vi "17_SoftwareClock.vi"() -> ()   [LabVIEW 2014]
uses:
  SwabianInstruments.TimeTagger
panel:
  out "SoftwareClockState":T1={"enabled"=FALSE, "is_locked"=FALSE, "period_error"=nan, "phase_error_estimation"=nan, "clock_period"=0, "error_counter"=0}
  in  "SoftwareClock settings":T2={"clock source"=enum."test signal as external clock", "input freq."=900000.0, "averaging_periods"=100.0, "trace_len"=1000, "clock channel"=1}
  in  "FrequencyStability settings":T3={"average"=1, "steps start"=1, "steps end"=100000, "number of steps"=100, "signal source"=enum."test signal", "signal channel"=2} {"number of steps" min=2 max=1000}
  out "Frequency error":T4(graph)
  out "Phase error":T5(graph)
  out "logger output":string="########################\n\nThis example demonstrates the SoftwareClock. The SoftwareClock is the recommended way to apply an external clock to the Time Tagger. Here, we will use the internal test signal for demonstration purposes. Be aware that this means decreasing the quality of the internal clock of your Time Tagger! If you have a high-quality external reference available, feel free to apply this and to set \"clock source\" to \"external clock\".\n\nThe settings of the SoftwareClock are updated every when the measurement is started.\n\nThe FrequencyStability measurement class provides numerous standard metrics conforming to IEEE 1139, e.g. the Allan Deviation (ADEV).\n\n########################\r\n\r\n"
  in  "exit":bool
  in  "run measurement":bool
  out "Time domain":cluster{"getTau":dbl[], "getHDEV":dbl[]}[](graph)
  out "Allan domain":cluster{"getTau":dbl[], "getSTDD":dbl[]}[](graph)
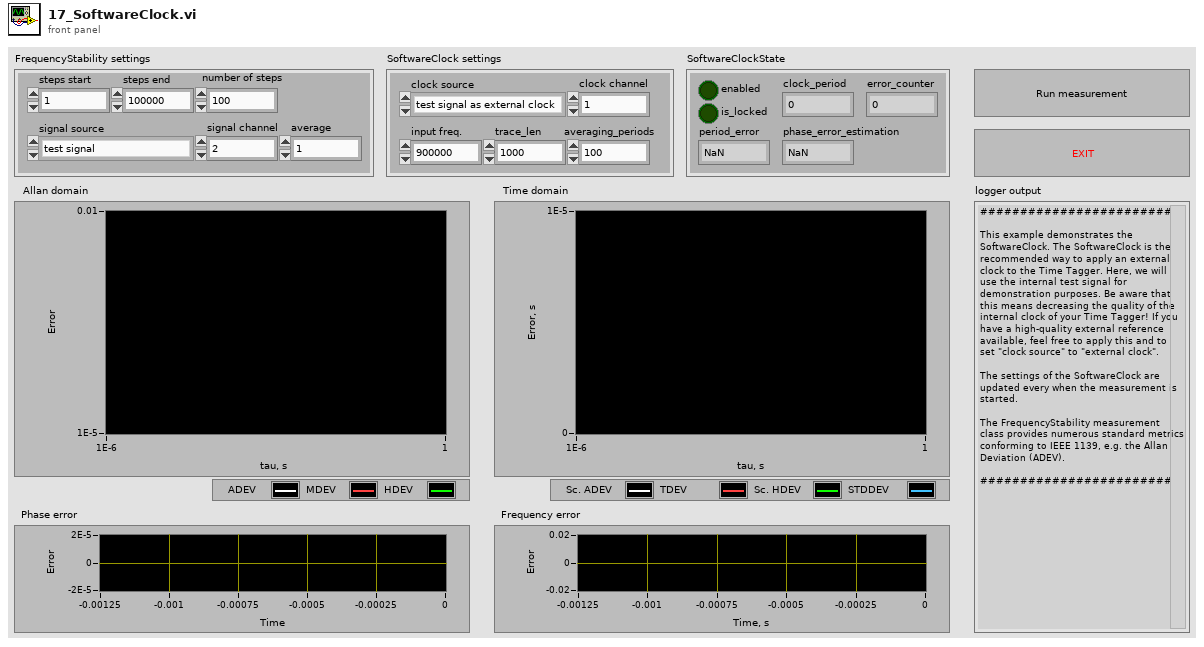
[diagram p1: front panel]
types:
  T1 = cluster{"enabled":bool, "is_locked":bool, "period_error":dbl, "phase_error_estimation":dbl, "clock_period":i64, "error_counter":i64}
  T2 = cluster{"clock source":enum16{"internal clock", "external clock", "test signal as external clock"}, "input freq.":dbl, "averaging_periods":dbl, "trace_len":u64, "clock channel":i32}
  T3 = cluster{"average":i64, "steps start":i32, "steps end":i32, "number of steps":i32, "signal source":enum16{"external signal", "test signal"}, "signal channel":i32}
  T4 = cluster{"getTraceIndex":dbl[], "getTraceFrequency":dbl[]}
  T5 = cluster{"getTraceIndex":dbl[], "getTracePhase":dbl[]}
  T6 = enum16{"internal clock", "external clock", "test signal as external clock"}
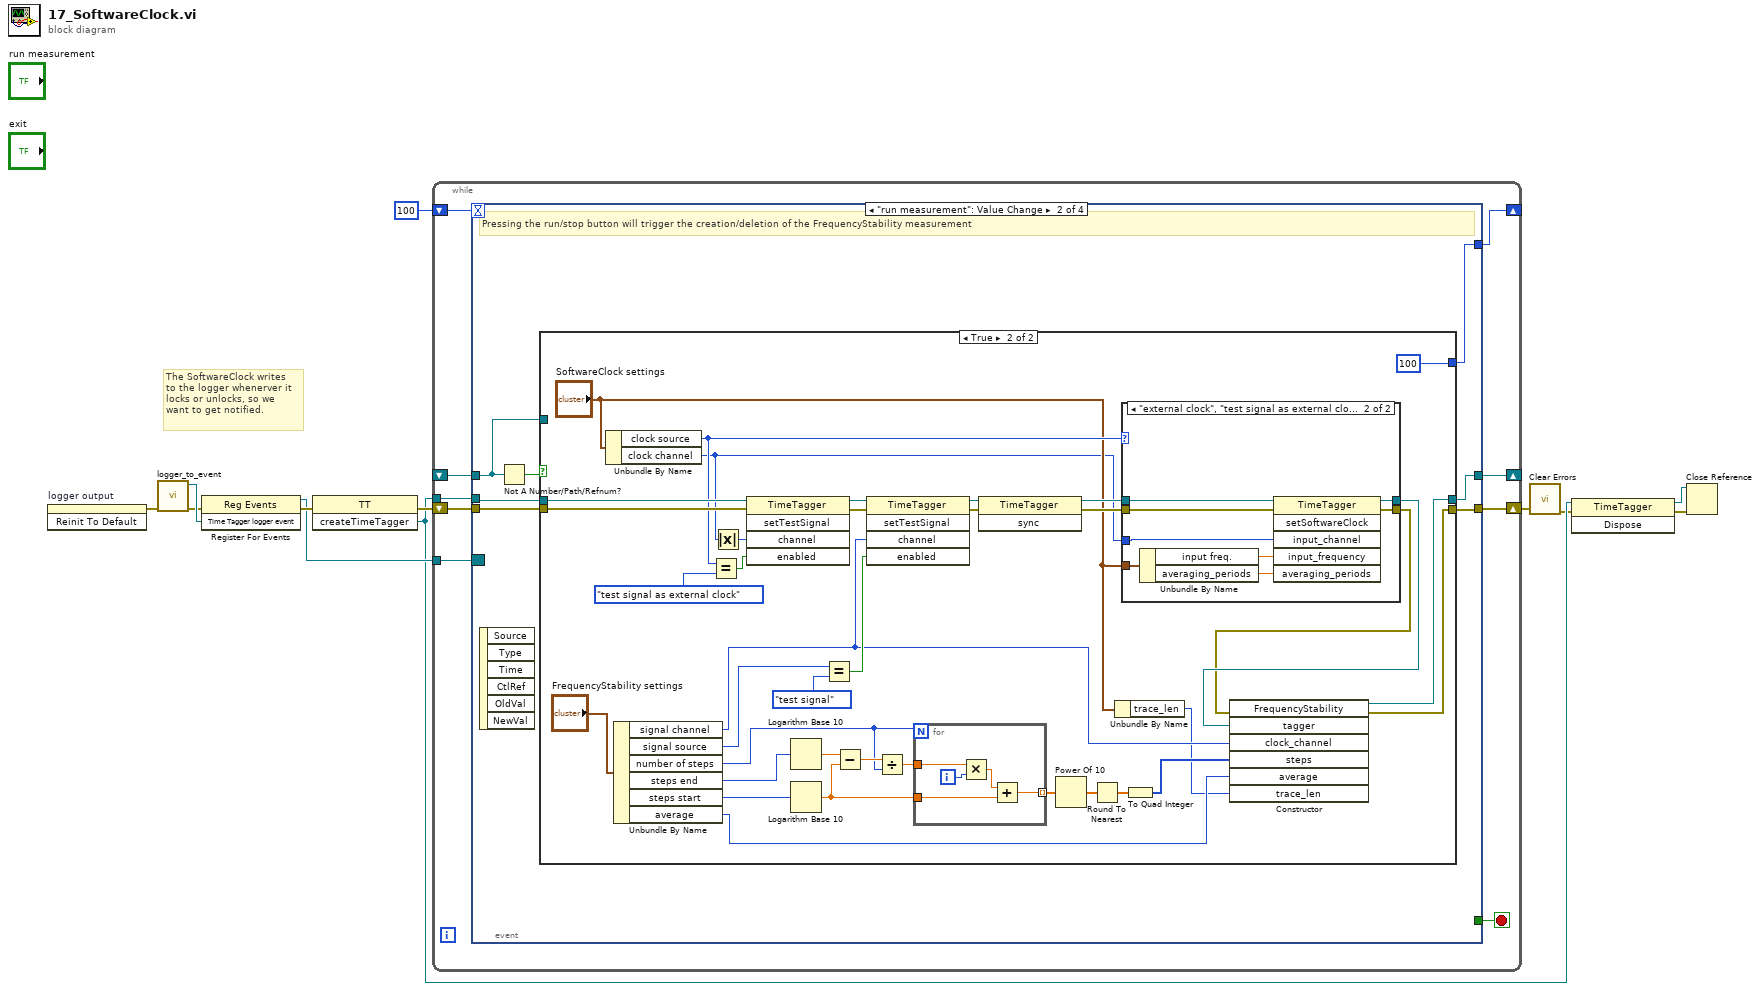
[diagram p0: block diagram]
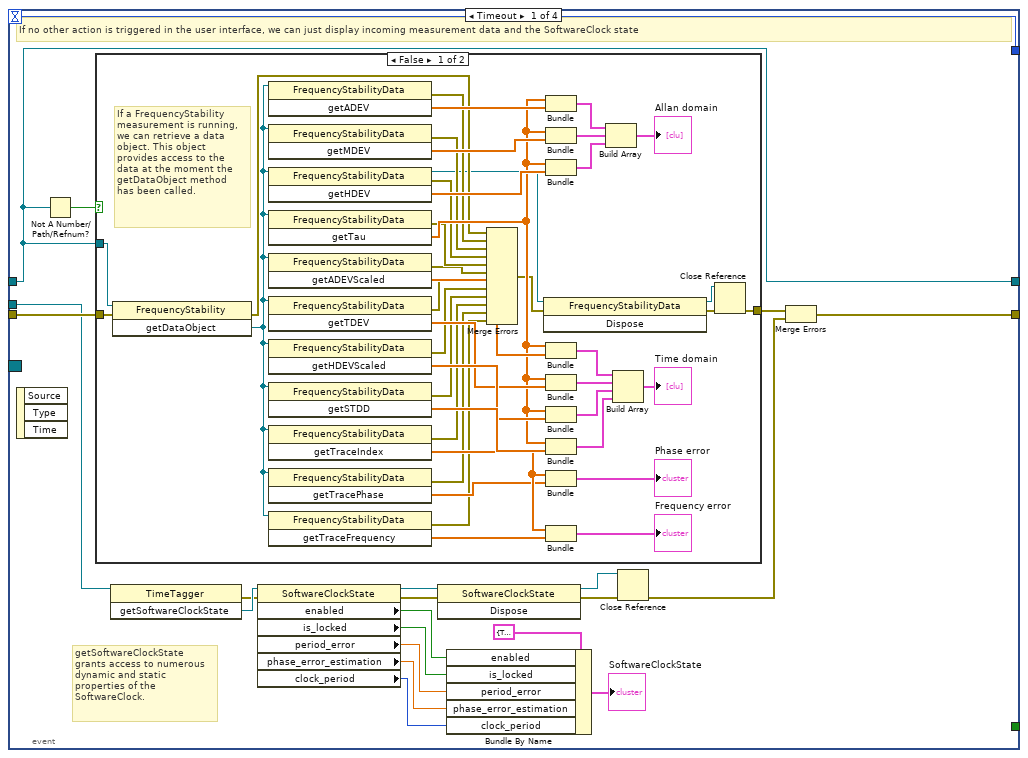
[diagram p2: hidden frame]
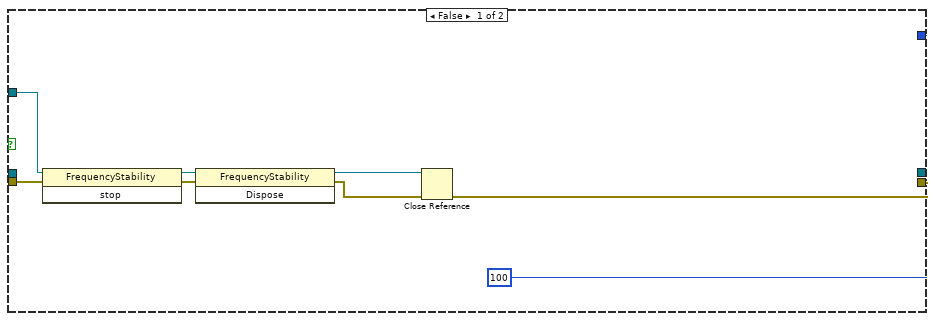
[diagram p4: hidden frame]
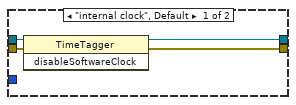
[diagram p5: hidden frame]
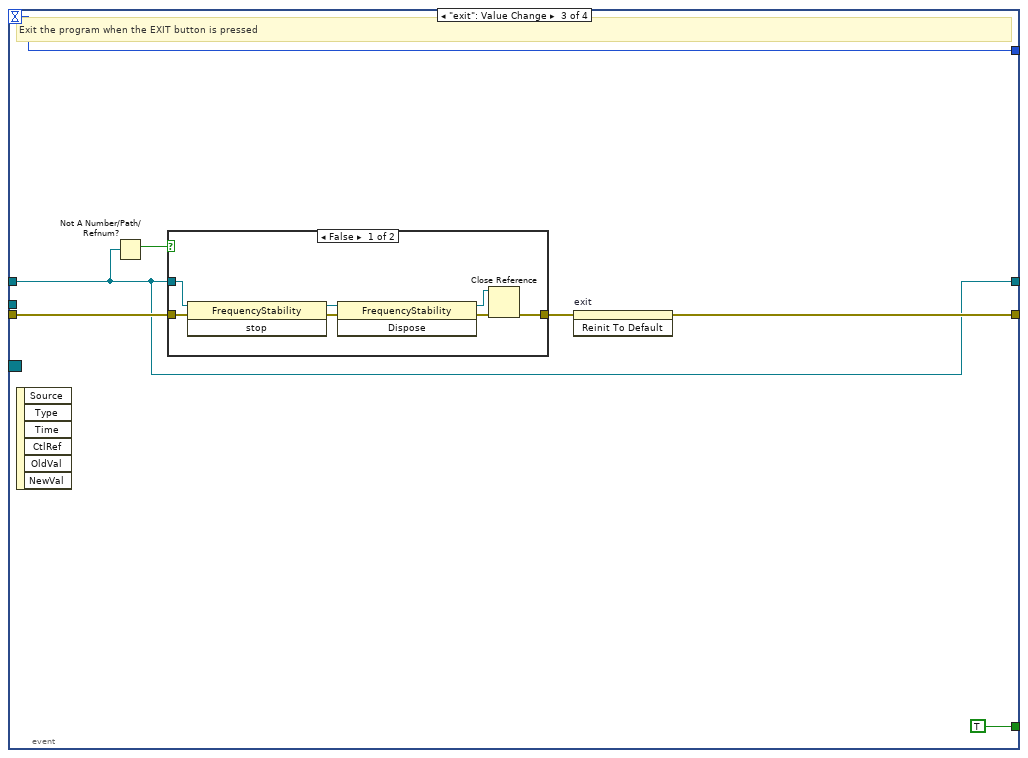
[diagram p6: hidden frame]
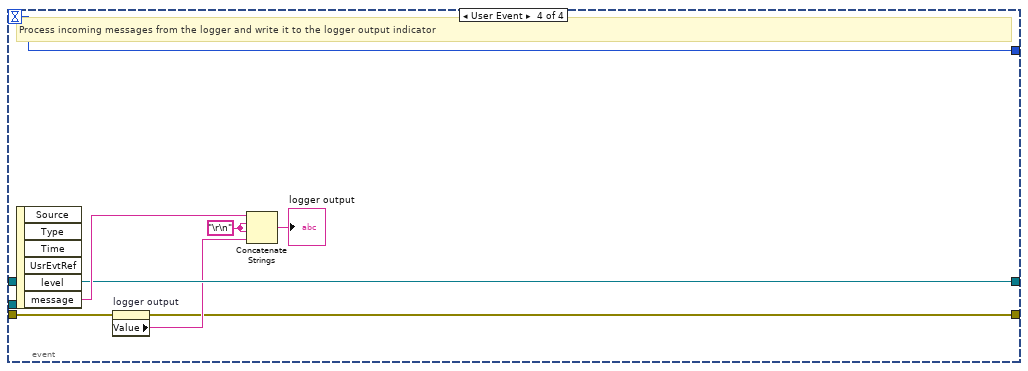
[diagram p8: hidden frame]
diagram:
  # "The SoftwareClock writes\nto the logger whenerver it\nlocks or unlocks, so we\nwant to get notified."
  n1 = invoke on="logger output" class="Str" method="Reinit To Default"() -> (error out=w6:errorcluster)  [unwired: 3 in, 2 out]
  n2 = call "logger_to_event.vi"("error in (no error)"=w6) -> ("error out"=w9:errorcluster, "Time Tagger logger event"=w10:refnum<user-event>)  [unwired: 9 in]
  n3 = register-events(error in=w9, w10) -> (reference out=w7:refnum<event-registration>, error out=w8:errorcluster)  [unwired: 1 in]
  n4 = invoke class="TT" method="createTimeTagger"(error in=w8) -> (error out=w11:errorcluster, "createTimeTagger"=w4:refnum<k24>)  [unwired: 2 in, 1 out]
  n5 = while {
    tunnel: w4 -> [w21]
    shift-right: [w20] -> _
    shift-left: _ -> [w19]
    shift-right: [w17] -> _
    shift-left: 100 -> [w18]
    shift-right: [w15] -> w5
    shift-left: w11 -> [w16]
    tunnel: w7 -> [w13]
    stop <- w14 stop-if-true
    n6 = event shown="[1] \"run measurement\": Value Change" {
      selector: w13 -> [_ _ _ _]
      dyn-events: _ -> [_ _ _ _]
      timeout: w18 -> [w25 _ w159 w175]
      tunnel: w21 -> [w40 w92 _ _]
      tunnel: [w42 w91 w155 w176] -> w20
      tunnel: w19 -> [w42 w89 w155 w176]
      tunnel: [w25 w88 w159 w175] -> w17
      tunnel: w16 -> [w41 w87 w156 w170]
      tunnel: [w23 w86 w161 w171] -> w15
      tunnel: [_ _ TRUE _] -> w14
      event Timeout {
        # "getSoftwareClockState\ngrants access to numerous\ndynamic and static\nproperties of the\nSoftwareClock."
        # "If no other action is triggered in the user interface, we can just display incoming measurement data and the SoftwareClock state"
        n7 = event-data() -> ()  [unwired: 1 in, 3 out]
        n8 = Not A Number/Path/Refnum?(number/path/refnum=w42) -> (NaN/Path/Refnum?=w39:bool)
        n9 = case shown="False" w39 {
          tunnel: w42 -> [w84 _]
          tunnel: w41 -> [w83 w85]
          tunnel: [w61 w85] -> w24
          frame False {
            # "If a FrequencyStability\nmeasurement is running,\nwe can retrieve a data\nobject. This object\nprovides access to the\ndata at the moment the\ngetDataObject method\nhas been called."
            n10 = invoke class="FrequencyStability" method="getDataObject"(reference=w84, error in=w83) -> (error out=w65:errorcluster, "getDataObject"=w60:refnum<k24>)  [unwired: 1 in, 1 out]
            n11 = invoke class="FrequencyStabilityData" method="getADEV"(reference=w60) -> (error out=w54:errorcluster, "getADEV"=w82:dbl[])  [unwired: 2 in, 1 out]
            n12 = invoke class="FrequencyStabilityData" method="getMDEV"(reference=w60) -> (error out=w53:errorcluster, "getMDEV"=w81:dbl[])  [unwired: 2 in, 1 out]
            n13 = invoke class="FrequencyStabilityData" method="getHDEV"(reference=w60) -> (reference out=w43:refnum<k24>, error out=w52:errorcluster, "getHDEV"=w80:dbl[])  [unwired: 2 in]
            n14 = invoke class="FrequencyStabilityData" method="getTau"(reference=w60) -> (error out=w51:errorcluster, "getTau"=w75:dbl[])  [unwired: 2 in, 1 out]
            n15 = invoke class="FrequencyStabilityData" method="getADEVScaled"(reference=w60) -> (error out=w50:errorcluster, "getADEVScaled"=w76:dbl[])  [unwired: 2 in, 1 out]
            n16 = invoke class="FrequencyStabilityData" method="getTDEV"(reference=w60) -> (error out=w49:errorcluster, "getTDEV"=w77:dbl[])  [unwired: 2 in, 1 out]
            n17 = invoke class="FrequencyStabilityData" method="getHDEVScaled"(reference=w60) -> (error out=w48:errorcluster, "getHDEVScaled"=w78:dbl[])  [unwired: 2 in, 1 out]
            n18 = invoke class="FrequencyStabilityData" method="getSTDD"(reference=w60) -> (error out=w47:errorcluster, "getSTDD"=w79:dbl[])  [unwired: 2 in, 1 out]
            n19 = invoke class="FrequencyStabilityData" method="getTraceIndex"(reference=w60) -> (error out=w46:errorcluster, "getTraceIndex"=w58:dbl[])  [unwired: 2 in, 1 out]
            n20 = invoke class="FrequencyStabilityData" method="getTracePhase"(reference=w60) -> (error out=w45:errorcluster, "getTracePhase"=w57:dbl[])  [unwired: 2 in, 1 out]
            n21 = invoke class="FrequencyStabilityData" method="getTraceFrequency"(reference=w60) -> (error out=w44:errorcluster, "getTraceFrequency"=w59:dbl[])  [unwired: 2 in, 1 out]
            n22 = Merge Errors(w65, w54, w53, w52, w51, w50, w49, w48, w47, w46, w45, w44) -> (w64:errorcluster)
            n23 = invoke class="FrequencyStabilityData" method="Dispose"(reference=w43, error in=w64) -> (reference out=w63:refnum<k24>, error out=w62:errorcluster)  [unwired: 1 in, 1 out]
            n24 = Bundle("getTau"=w75, "getADEV"=w82) -> (w74:cluster{"getTau":dbl[], "getADEV":dbl[]})  [unwired: 1 in]
            n25 = Bundle("getTau"=w75, "getMDEV"=w81) -> (w73:cluster{"getTau":dbl[], "getMDEV":dbl[]})  [unwired: 1 in]
            n26 = Bundle("getTau"=w75, "getHDEV"=w80) -> (w72:cluster{"getTau":dbl[], "getHDEV":dbl[]})  [unwired: 1 in]
            n27 = Bundle("getTau"=w75, "getADEVScaled"=w76) -> (w71:cluster{"getTau":dbl[], "getADEVScaled":dbl[]})  [unwired: 1 in]
            n28 = Bundle("getTau"=w75, "getTDEV"=w77) -> (w70:cluster{"getTau":dbl[], "getTDEV":dbl[]})  [unwired: 1 in]
            n29 = Bundle("getTau"=w75, "getHDEVScaled"=w78) -> (w69:cluster{"getTau":dbl[], "getHDEVScaled":dbl[]})  [unwired: 1 in]
            n30 = Bundle("getTau"=w75, "getSTDD"=w79) -> (w68:cluster{"getTau":dbl[], "getSTDD":dbl[]})  [unwired: 1 in]
            n31 = Bundle("getTraceIndex"=w58, "getTracePhase"=w57) -> (→"Phase error":T5)  [unwired: 1 in]
            n32 = Bundle("getTraceIndex"=w58, "getTraceFrequency"=w59) -> (→"Frequency error":T4)  [unwired: 1 in]
            n33 = Build Array(w74, w73, w72) -> (→"Allan domain":cluster{"getTau":dbl[], "getHDEV":dbl[]}[])
            n34 = Build Array(w71, w70, w69, w68) -> (→"Time domain":cluster{"getTau":dbl[], "getSTDD":dbl[]}[])
            n35 = Close Reference(reference=w63, error in (no error)=w62) -> (error out=w61:errorcluster)
          }
          frame True {
          }
        }
        n36 = invoke class="TimeTagger" method="getSoftwareClockState"(reference=w40) -> (error out=w37:errorcluster, "getSoftwareClockState"=w38:refnum<k24>)  [unwired: 2 in, 1 out]
        n37 = property class="SoftwareClockState"(reference=w38, error in=w37) -> (reference out=w27:refnum<k24>, error out=w28:errorcluster, "enabled"=w36:bool, "is_locked"=w35:bool, "period_error"=w34:dbl, "phase_error_estimation"=w32:dbl, "clock_period"=w31:i64)
        n38 = invoke class="SoftwareClockState" method="Dispose"(reference=w27, error in=w28) -> (reference out=w30:refnum<k24>, error out=w29:errorcluster)  [unwired: 1 in, 1 out]
        n39 = Bundle By Name(cluster=T1 {"enabled"=TRUE, "is_locked"=TRUE, "period_error"=34575.234590264736, "phase_error_estimation"=8484.866795079515, "clock_period"=1111111, "error_counter"=1111111} ("SoftwareClockState"), "enabled"=w36, "is_locked"=w35, "period_error"=w34, "phase_error_estimation"=w32, "clock_period"=w31) -> (→"SoftwareClockState":T1)
        n40 = Close Reference(reference=w30, error in (no error)=w29) -> (error out=w22:errorcluster)
        n41 = Merge Errors(w24, w22) -> (w23:errorcluster)
      }
      event "run measurement": Value Change {
        # "Pressing the run/stop button will trigger the creation/deletion of the FrequencyStability measurement"
        n42 = event-data() -> ()  [unwired: 1 in, 6 out]
        n43 = Not A Number/Path/Refnum?(number/path/refnum=w89) -> (NaN/Path/Refnum?=w90:bool)
        n44 = case shown="True" w90 {
          tunnel: w92 -> [_ w116]
          tunnel: [_ w137] -> w91
          tunnel: w89 -> [w99 _]
          tunnel: [100 100] -> w88
          tunnel: w87 -> [w98 w129]
          tunnel: [w93 w124] -> w86
          frame False {
            n45 = invoke class="FrequencyStability" method="stop"(reference=w99, error in=w98) -> (reference out=w97:refnum<k24>, error out=w96:errorcluster)  [unwired: 1 in, 1 out]
            n46 = invoke class="FrequencyStability" method="Dispose"(reference=w97, error in=w96) -> (reference out=w95:refnum<k24>, error out=w94:errorcluster)  [unwired: 1 in, 1 out]
            n47 = Close Reference(reference=w95, error in (no error)=w94) -> (error out=w93:errorcluster)
          }
          frame True {
            n48 = Unbundle By Name("SoftwareClock settings") -> ("clock source"=w110:T6, "clock channel"=w106:i32)
            n49 = Unbundle By Name("FrequencyStability settings") -> ("signal channel"=w105:i32, "signal source"=w109:enum16{"external signal", "test signal"}, "number of steps"=w101:i32, "steps end"=w104:i32, "steps start"=w113:i32, "average"=w114:i64)
            n50 = Equal?(x=w110, y=T6."test signal as external clock") -> (x = y?=w111:bool)
            n51 = Absolute Value(x=w106) -> (abs(x)=w112:i32)
            n52 = invoke class="TimeTagger" method="setTestSignal"(reference=w116, error in=w129, "channel"=w112, "enabled"=w111) -> (reference out=w127:refnum<k24>, error out=w128:errorcluster)  [unwired: 1 in, 3 out]
            n53 = Logarithm Base 10(1:w104) -> (0:w134:dbl)
            n54 = Logarithm Base 10(1:w113) -> (0:w102:dbl)
            n55 = Equal?(x=w109, y=enum16{"external signal", "test signal"}."test signal") -> (x = y?=w118:bool)
            n56 = Subtract(x=w134, y=w102) -> (x-y=w136:dbl)
            n57 = invoke class="TimeTagger" method="setTestSignal"(reference=w127, error in=w128, "channel"=w105, "enabled"=w118) -> (reference out=w123:refnum<k24>, error out=w121:errorcluster)  [unwired: 1 in, 3 out]
            n58 = Divide(x=w136, y=w101) -> (x/y=w135:dbl)
            n59 = for {
              N: w101 -> [_]
              tunnel: w135 -> [w154]
              tunnel: [w151] -> w133 mode=indexing
              tunnel: w102 -> [w150]
              i -> [w153]
              n60 = Multiply(x=w154, y=w153) -> (x*y=w152:dbl)
              n61 = Add(x=w152, y=w150) -> (x+y=w151:dbl)
            }
            n62 = invoke class="TimeTagger" method="sync"(reference=w123, error in=w121) -> (reference out=w122:refnum<k24>, error out=w120:errorcluster)  [unwired: 1 in, 1 out]
            n63 = Power Of 10(x=w133) -> (10^x=w132:dbl[])
            n64 = Round To Nearest(number=w132) -> (nearest integer value=w131:dbl[])
            n65 = Unbundle By Name("SoftwareClock settings") -> ("trace_len"=w103:u64)
            n66 = case shown="\"external clock\", \"test signal as external clock\"" w110 {
              tunnel: [w138 w149] -> w126
              tunnel: [w139 w148] -> w125
              tunnel: w106 -> [_ w147]
              tunnel: w122 -> [w141 w146]
              tunnel: w120 -> [w140 w145]
              tunnel: "SoftwareClock settings" -> [_ w144]
              frame "internal clock", Default {
                n67 = invoke class="TimeTagger" method="disableSoftwareClock"(reference=w141, error in=w140) -> (reference out=w138:refnum<k24>, error out=w139:errorcluster)  [unwired: 1 in, 1 out]
              }
              frame "external clock", "test signal as external clock" {
                n68 = Unbundle By Name(w144) -> ("input freq."=w143:dbl, "averaging_periods"=w142:dbl)
                n69 = invoke class="TimeTagger" method="setSoftwareClock"(reference=w146, error in=w145, "input_channel"=w147, "input_frequency"=w143, "averaging_periods"=w142) -> (reference out=w149:refnum<k24>, error out=w148:errorcluster)  [unwired: 1 in, 4 out]
              }
            }
            n70 = To Quad Integer(1:w131) -> (0:w130:i64[])
            n71 = constructor class="FrequencyStability"(error in=w125, "tagger"=w126, "clock_channel"=w105, "steps"=w130, "average"=w114, "trace_len"=w103) -> (reference out=w137:refnum<k24>, error out=w124:errorcluster)  [unwired: 2 in, 6 out]
          }
        }
      }
      event "exit": Value Change {
        # "Exit the program when the EXIT button is pressed"
        n72 = event-data() -> ()  [unwired: 1 in, 6 out]
        n73 = Not A Number/Path/Refnum?(number/path/refnum=w155) -> (NaN/Path/Refnum?=w158:bool)
        n74 = case shown="False" w158 {
          tunnel: w155 -> [w163 _]
          tunnel: [w164 w169] -> w157
          tunnel: w156 -> [w162 w169]
          frame False {
            n75 = invoke class="FrequencyStability" method="stop"(reference=w163, error in=w162) -> (reference out=w168:refnum<k24>, error out=w167:errorcluster)  [unwired: 1 in, 1 out]
            n76 = invoke class="FrequencyStability" method="Dispose"(reference=w168, error in=w167) -> (reference out=w166:refnum<k24>, error out=w165:errorcluster)  [unwired: 1 in, 1 out]
            n77 = Close Reference(reference=w166, error in (no error)=w165) -> (error out=w164:errorcluster)
          }
          frame True {
          }
        }
        n78 = invoke on="exit" class="Bool" method="Reinit To Default"(error in=w157) -> (error out=w161:errorcluster)  [unwired: 2 in, 2 out]
      }
      event User Event {
        w174 = "\r\n"
        # "Process incoming messages from the logger and write it to the logger output indicator"
        n79 = event-data() -> ("message"=w177:string)  [unwired: 1 in, 5 out]
        n80 = property on="logger output" class="Str"(error in=w170) -> (error out=w171:errorcluster, "Value"=w173:string)  [unwired: 1 in, 1 out]
        n81 = Concatenate Strings(w177, w174, w174, w173) -> (→"logger output":string)
      }
    }
  }
  n82 = call <vilib>:"Clear Errors.vi"("error in (no error)"=w5) -> ("error out"=w1:errorcluster)  [unwired: 5 in, 1 out]
  n83 = invoke class="TimeTagger" method="Dispose"(reference=w4, error in=w1) -> (reference out=w2:refnum<k24>, error out=w3:errorcluster)  [unwired: 1 in, 1 out]
  n84 = Close Reference(reference=w2, error in (no error)=w3) -> ()  [unwired: 1 out]
